vi "LinearSystemLoop_GetU.vi"(11 "input inear System Loop":T1) -> (3 "U":T3)   [LabVIEW 2019, in "Trajectory_Library.lvlib"]
doc: "Returns the controller's calculated control input u plus the calculated feedforward u_ff.\n \nInputs:\n - LinearSystemLoop -- system data cluster\n\nOutputs:\n - U -- the calculated control input u."
uses:
  Trajectory_Library.lvlib
  <vilib>/Analysis/Matrix/Datatypes/RealMatrix.ctl
  LINEAR_SYSTEM_LOOP.ctl
  LINEAR_QUADRATIC_REGULATOR.ctl
  LINEAR_PLANT_INV_FF.ctl
  KALMAN_FILTER.ctl
  LINEAR_SYSTEM.ctl
  <vilib>/Analysis/Matrix/Numeric/Add/Add - RM,RM.vi
  <vilib>/Analysis/Matrix/NI_Matrix.lvlib
panel:
  # "<States,1>"
  # "<FUTURE --- CLAMP TYPE -- For now\nuse Normalize>"
  # "Steady State Gain  \n<States,Outputs>"
  # "State Estimate <Statess,1>"
  # "<States,States>"
  # "<States,Inputs>"
  # "<Outputs,States>"
  # "<Outputs,Inputs>"
  # "<States,1>"
  # "<Inputs,1>"
  # "<States,Inputs>"
  # "<States,States>"
  # "Ref State <States,1>"
  # "Comp and capped \noutput <Inputs,1>"
  # "Controller gain\n<Inputs,States>"
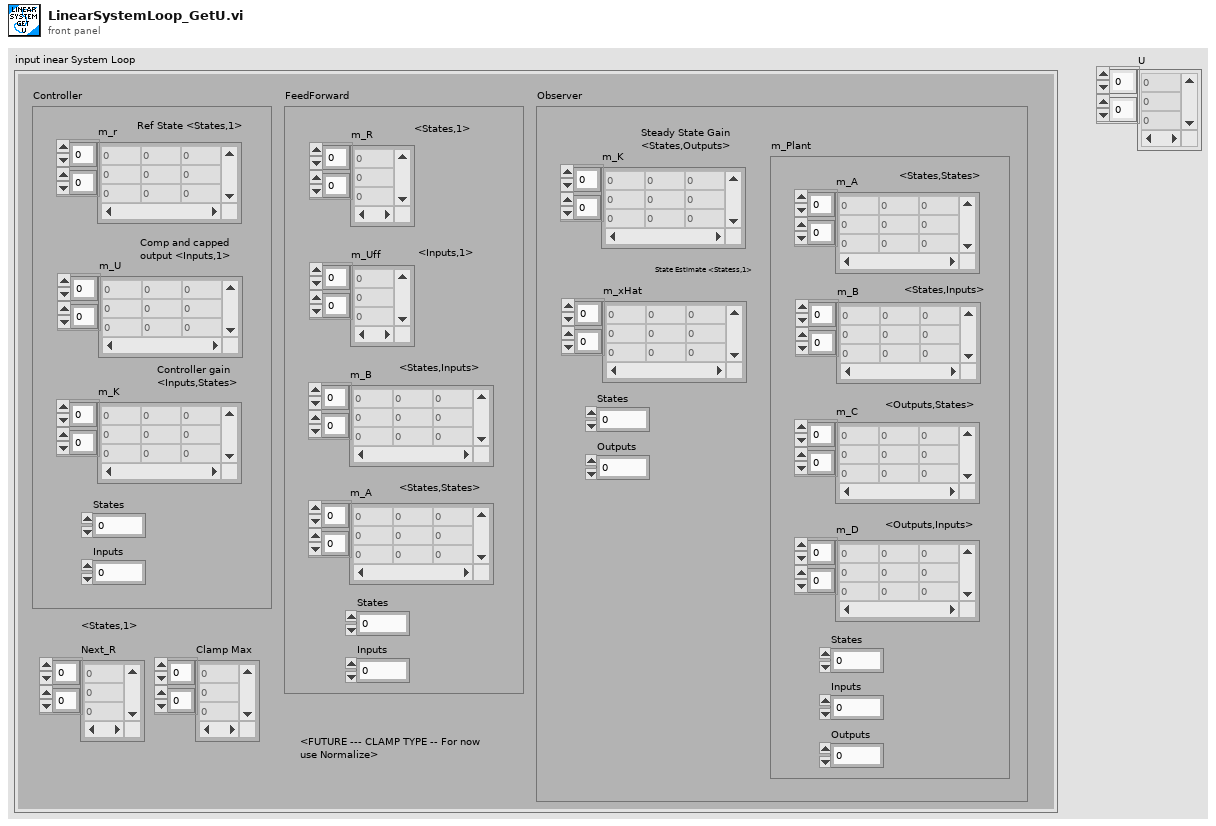
[diagram p1: front panel]
types:
  T1 = typedef "Trajectory_Library.lvlib/LINEAR_SYSTEM_LOOP.ctl" = cluster{"Controller":T2, "FeedForward":T4, "Observer":T5, "Next_R":T3, "Clamp Max":T3}
  T2 = typedef "Trajectory_Library.lvlib/LINEAR_QUADRATIC_REGULATOR.ctl" = cluster{"m_r":T3, "m_U":T3, "m_K":T3, "States":i32, "Inputs":i32}
  T3 = typedef "NI_Matrix.lvlib/RealMatrix.ctl" = dbl[][]
  T4 = typedef "Trajectory_Library.lvlib/LINEAR_PLANT_INV_FF.ctl" = cluster{"m_R":T3, "m_Uff":T3, "m_B":T3, "m_A":T3, "States":i32, "Inputs":i32}
  T5 = typedef "Trajectory_Library.lvlib/KALMAN_FILTER.ctl" = cluster{"m_K":T3, "m_xHat":T3, "States":i32, "Outputs":i32, "m_Plant":T6}
  T6 = typedef "Trajectory_Library.lvlib/LINEAR_SYSTEM.ctl" = cluster{"m_A":T3, "m_B":T3, "m_C":T3, "m_D":T3, "States":i32, "Inputs":i32, "Outputs":i32}
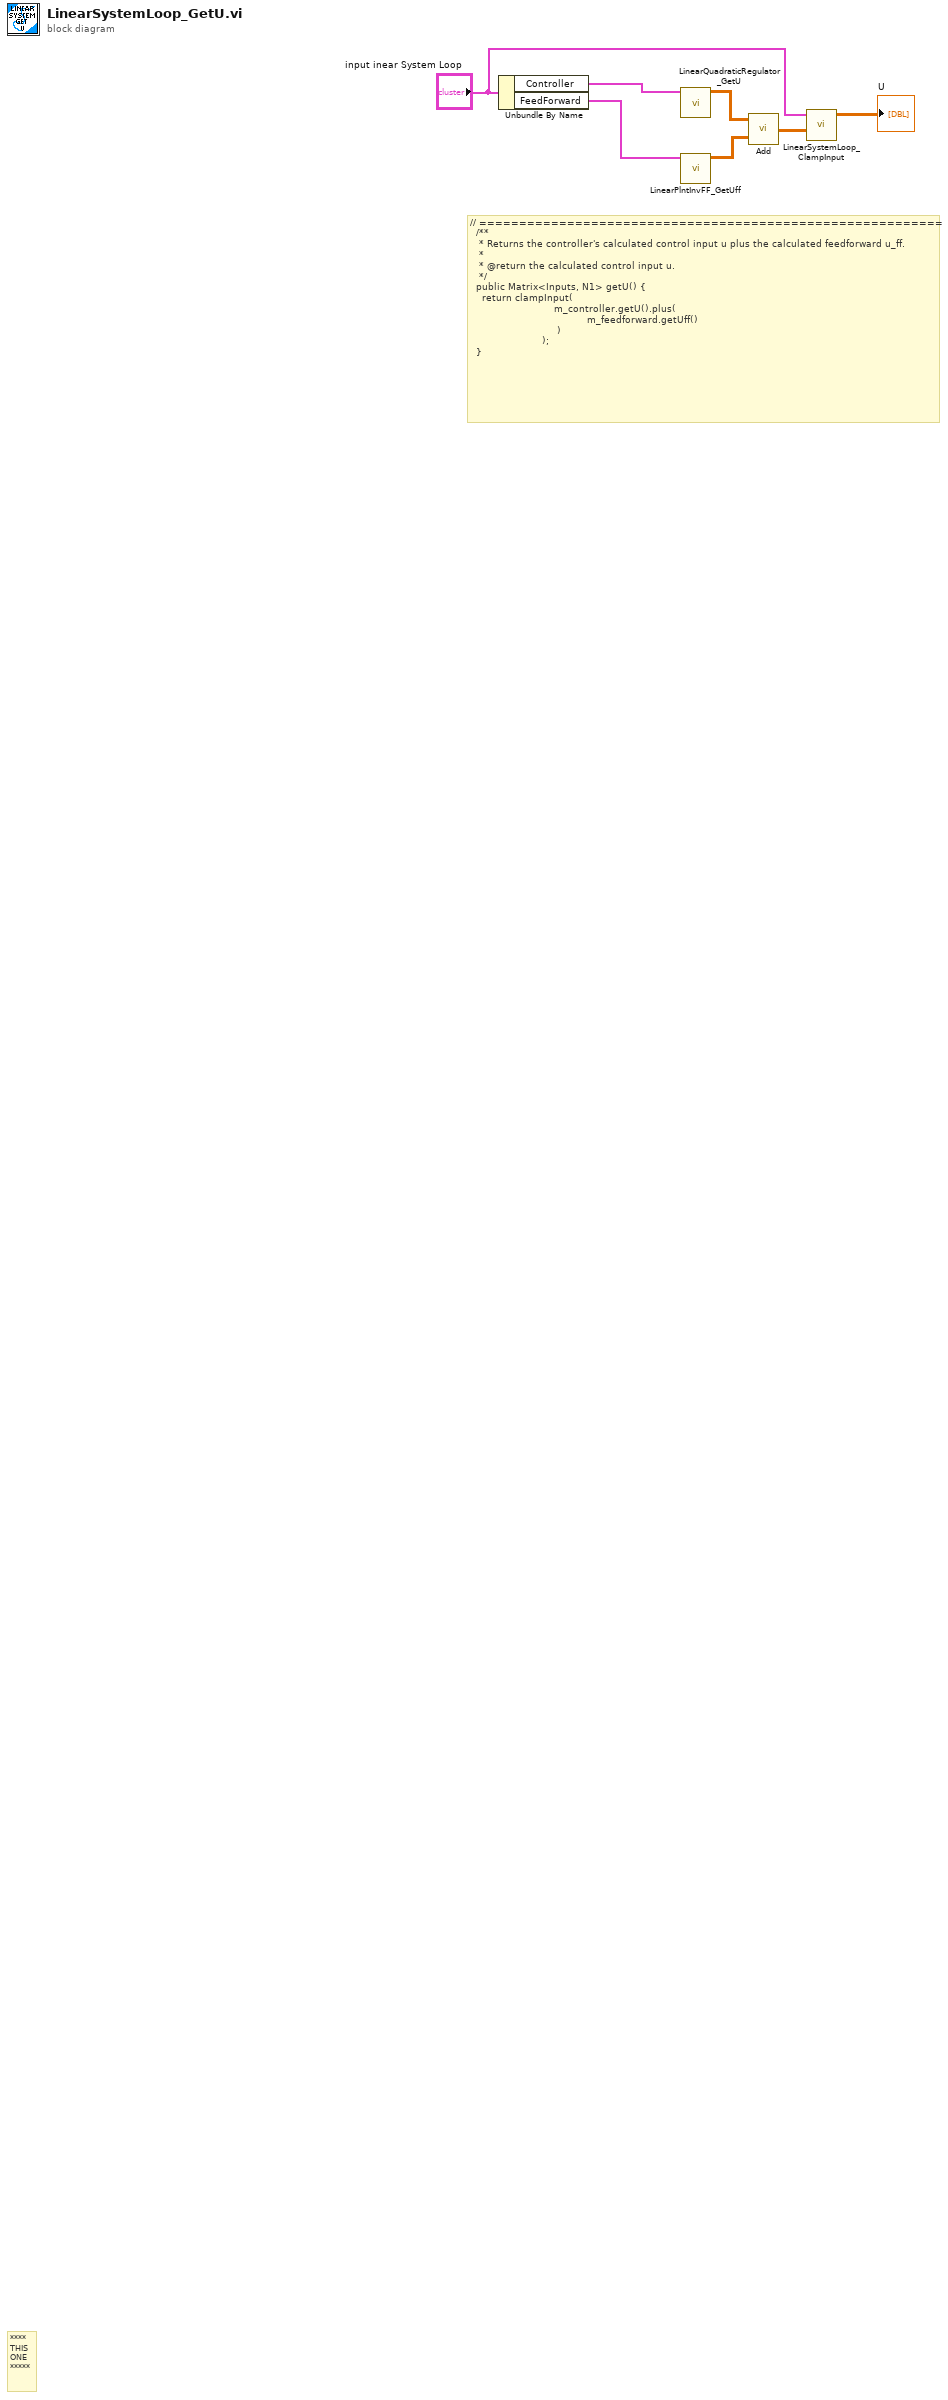
[diagram p0: block diagram]
diagram:
  # "// ==========================================================\n  /**\n   * Returns the controller's calculated control input u plus the calculated feedforward u_ff.\n   *\n   * @return the calculated control input u.\n   */\n  public Matrix<Inputs, N1> getU() {\n    return clampInput(\n                            m_controller.getU().plus( \n                                       m_feedforward.getUff() \n                             )\n                        );\n  }"
  # "****\nTHIS\nONE\n*****"
  n1 = Unbundle By Name("input inear System Loop") -> ("Controller"=w7:T2, "FeedForward"=w6:T4)
  n2 = call "LinearQuadraticRegulator_GetU.vi"("in LinearQuadraticRegulator"=w7) -> ("U"=w5:T3)  [unwired: 10 in]
  n3 = call "LinearPlntInvFF_GetUff.vi"("Linear Plnt Inversion FF"=w6) -> ("Uff"=w4:T3)  [unwired: 10 in]
  n4 = call-poly <vilib>:"Add.vi"("Real Matrix B"=w4, "Real Matrix A"=w5) -> ("A + B"=w2:T3)
  n5 = call "LinearSystemLoop_ClampInput.vi"("UnclampedU"=w2, "input inear System Loop"="input inear System Loop") -> ("U"=→"U":T3)  [unwired: 8 in, 1 out]
